vi "Send Trigger.vi"(8 "error in (no error)":errorcluster, 9 "Mode (0: Sweep)":u16(ring) items=["Sweep", "Burst"], 10 "Channel (1:Channel 1)":i32(ring)=1 items=["Channel 1"=1, "Channel 2"=2], 11 "VISA resource name":refnum<visa-resource-name>) -> (0 "error out":errorcluster, 3 "VISA resource name out":refnum<visa-resource-name>)   [LabVIEW 2015, in "SDG X Series.lvlib"]
doc: "Sends a command to the selected channel that simulates a front panel manual trigger to the instrument. You can use this vi to trigger a frequency sweep or burst output. You must first set Trigger Source to Manual in <b>Configure Frequency Sweep.vi</b> or <b>Configure Burst Output.vi</b> respectively.\n\n<B>Note: </B> Use this VI only with other low-level VIs."
uses:
  <instrlib>/SDG X Series/SDG X Series.lvlib
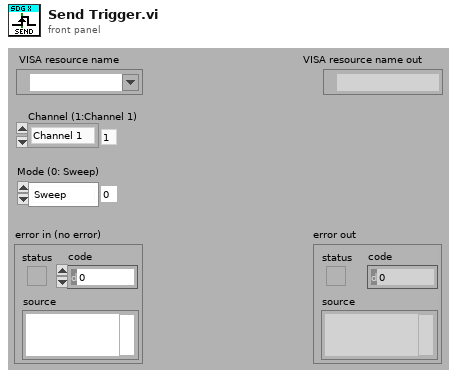
[diagram p1: front panel]
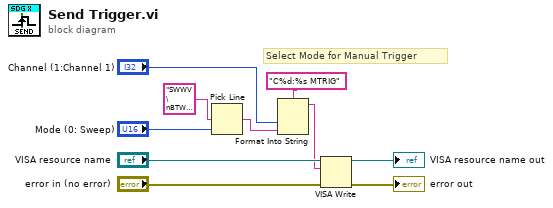
[diagram p0: block diagram]
diagram:
  # "Select Mode for Manual Trigger"
  n1 = Pick Line(multi-line string="SWWV\nBTWV", line index="Mode (0: Sweep)") -> (output string=w2:string)  [unwired: 1 in]
  n2 = Format Into String(format string="C%d:%s MTRIG", "Channel (1:Channel 1)", w2) -> (resulting string=w4:string)  [unwired: 2 in, 1 out]
  n3 = VISA Write(VISA resource name="VISA resource name", write buffer=w4, error in (no error)="error in (no error)") -> (VISA resource name out=→"VISA resource name out":refnum<visa-resource-name>, error out=→"error out":errorcluster)  [unwired: 1 out]
